vi "Do.vi"(8 "error in (no error)":errorcluster, 10 "Actor in":refnum<class "Actor.lvclass">, 11 "Add Wfm Header Msg":refnum<class "Add Wfm Header Msg.lvclass">) -> (0 "error out":errorcluster, 2 "Actor out":refnum<class "Actor.lvclass">)   [LabVIEW 2012, in "TCP Classes.lvlib" / "Add Wfm Header Msg.lvclass"]
doc: "This VI delivers the message to the actor by calling the appropriate method(s) on the actor."
uses:
  Add Wfm Header Msg.lvclass
  <vilib>/ActorFramework/Actor/Actor.lvclass
  Class TCP Writer/TCP Writer.lvclass
  Add Wfm Header Msg.lvclass/Add Wfm Header Msg.ctl
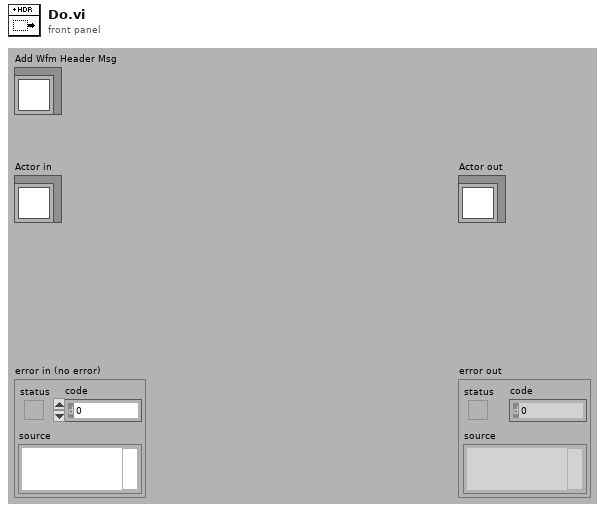
[diagram p1: front panel]
types:
  T1 = typedef "Waveform Header.ctl" = cluster{"dt":dbl, "attributes (str)":string[][]}
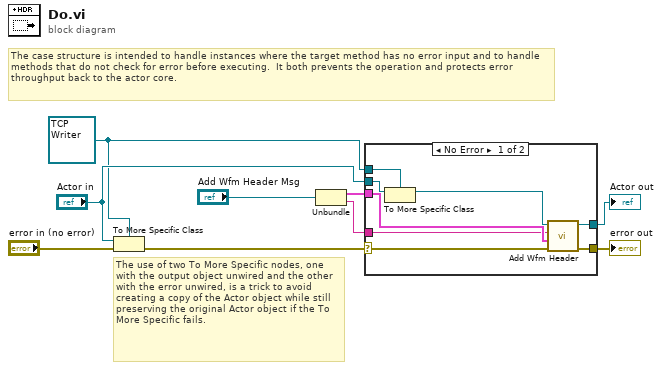
[diagram p0: block diagram]
diagram:
  w3 = refnum<class "TCP Writer.lvclass"> refnum ("Actor in")
  # "The use of two To More Specific nodes, one with the output object unwired and the other with the error unwired, is a trick to avoid creating a copy of the Actor object while still preserving the original Actor object if the To More Specific fails."
  # "The case structure is intended to handle instances where the target method has no error input and to handle methods that do not check for error before executing.  It both prevents the operation and protects error throughput back to the actor core."
  n1 = To More Specific Class(target class=w3, reference="Actor in", error in="error in (no error)") -> (error out=w7:errorcluster)  [unwired: 1 out]
  n2 = Unbundle("Add Wfm Header Msg") -> (w2:T1, w1:string)
  n3 = case shown="No Error" w7 {
    selector: w7 -> [w15 w19]
    tunnel: [w17 w19] -> w6
    tunnel: [w16 w18] -> w5
    tunnel: "Actor in" -> [w14 w18]
    tunnel: w3 -> [w13 _]
    tunnel: w2 -> [w11 _]
    tunnel: w1 -> [w10 _]
    frame No Error {
      n4 = To More Specific Class(target class=w13, reference=w14) -> (specific class reference=w12:refnum<class "TCP Writer.lvclass">)  [unwired: 1 in, 1 out]
      n5 = call "Add Wfm Header.vi"("error in (no error)"=w15, "Wfm Header"=w11, "Metadata"=w10, "TCP Writer in"=w12) -> ("error out"=w17:errorcluster, "TCP Writer out"=w16:refnum<class "TCP Writer.lvclass">)  [unwired: 6 in]
    }
    frame Error {
      # "If type check fails, pass the original object out again."
    }
  }
  "error out" <- w6
  "Actor out" <- w5
